vi "RunRotation.vi"(8 "error in (no error)":errorcluster, 11 "Microscope in":refnum<class "Microscope.lvclass">) -> (0 "error out":errorcluster, 3 "Microscope out":refnum<class "Microscope.lvclass">)   [LabVIEW 2012, in "Microscope.lvclass"]
uses:
  classes/Microscope.lvclass
  classes/Microscope.lvclass/Microscope.ctl
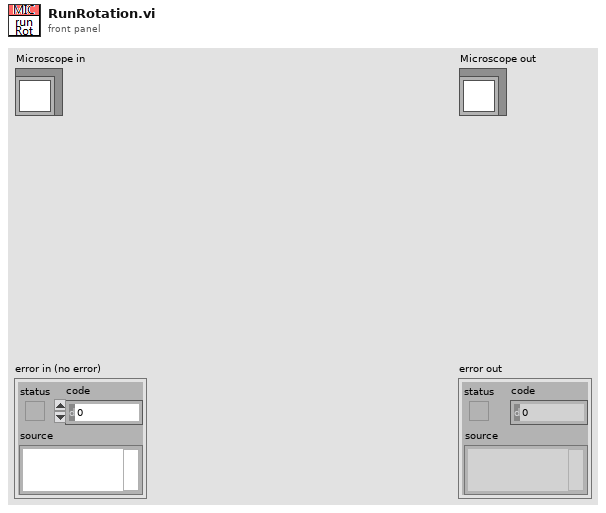
[diagram p1: front panel]
types:
  T1 = enum32{"Invalid", "Standard", "Closed", "Hidden", "Minimized", "Maximized"}
  T2 = typedef "ScanMode.ctl" = enum16{"None", "Continuous", "Point Scan (CH3 cursor)", "Point Scan Move (CH3 cursor)", "Grab", "Grab Move Stage", "Grab Move Z-stage", "Cont. Move Z-stage", "Spec Move Stage", "Spec Move Cont", "Surf Calib"}
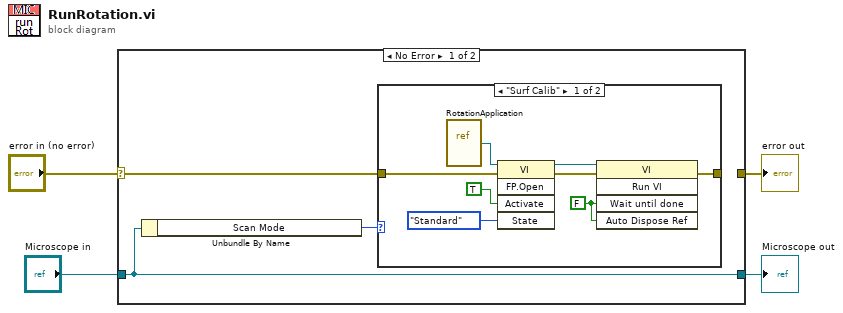
[diagram p0: block diagram]
diagram:
  n1 = case shown="No Error" "error in (no error)" {
    selector: "error in (no error)" -> [w5 w18]
    tunnel: [_ w18] -> w3
    tunnel: [w7 w17] -> w1
    tunnel: "Microscope in" -> [w7 w17]
    frame No Error {
      n2 = Unbundle By Name(w7) -> ("Scan Mode"=w6:T2)
      n3 = case shown="\"Surf Calib\"" w6 {
        tunnel: [w10 w16] -> _
        tunnel: w5 -> [w8 w16]
        frame "Surf Calib" {
          w9 = FALSE ("Wait Until Done")
          n4 = vi-ref "RotationApplication.vi"() -> (w13:refnum<vi>)
          n5 = invoke class="VI" method="FP.Open"(reference=w13, error in=w8, "Activate"=TRUE ("Activate?"), "State"=T1."Standard") -> (reference out=w12:refnum<vi>, error out=w11:errorcluster)  [unwired: 1 in, 3 out]
          n6 = invoke class="VI" method="Run VI"(reference=w12, error in=w11, "Wait until done"=w9, "Auto Dispose Ref"=w9) -> (error out=w10:errorcluster)  [unwired: 1 in, 4 out]
        }
        frame "None", Default {
        }
      }
    }
    frame Error {
    }
  }
  "error out" <- w3
  "Microscope out" <- w1
